vi "initBoardAllInOne.vi"(5 "On Sum\nOff Majority":bool=TRUE, 8 "error in (no error)":errorcluster, 10 "address":string="172.16.7.43", 11 "remote port or service name":u16=9764) -> (0 "error out":errorcluster)   [LabVIEW 2009]
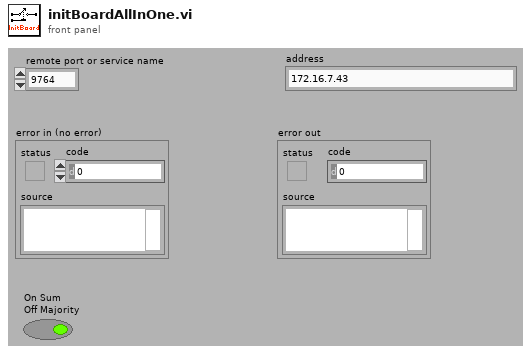
[diagram p1: front panel]
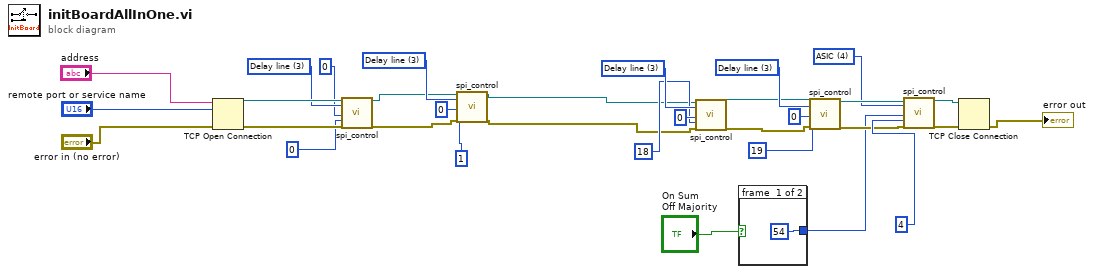
[diagram p0: block diagram]
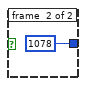
[diagram p2: hidden frame]
diagram:
  w11 = u16 4 items=["Attenuation", "Clipping", "Enable channel", "Delay line", "ASIC"] ("Device")
  w19 = u16 3 items=["Attenuation", "Clipping", "Enable channel", "Delay line", "ASIC"] ("Device")
  w22 = u16 3 items=["Attenuation", "Clipping", "Enable channel", "Delay line", "ASIC"] ("Device")
  w25 = u16 3 items=["Attenuation", "Clipping", "Enable channel", "Delay line", "ASIC"] ("Device")
  w28 = u16 3 items=["Attenuation", "Clipping", "Enable channel", "Delay line", "ASIC"] ("Device")
  n1 = TCP Open Connection(address="address", remote port or service name="remote port or service name", error in (no error)="error in (no error)") -> (connection ID=w29:refnum<k5>, error out=w30:errorcluster)  [unwired: 2 in]
  n2 = call "spi_control.vi"("connection ID"=w29, "Device"=w28, "Data"=0, "Register or channel"=0, "error out 3"=w30) -> ("connection ID out"=w16:refnum<k5>, "error out 2"=w15:errorcluster)  [unwired: 7 in, 6 out]
  n3 = call "spi_control.vi"("connection ID"=w16, "Device"=w25, "Data"=0, "Register or channel"=1, "error out 3"=w15) -> ("connection ID out"=w4:refnum<k5>, "error out 2"=w3:errorcluster)  [unwired: 7 in, 6 out]
  n4 = call "spi_control.vi"("connection ID"=w4, "Device"=w22, "Data"=0, "Register or channel"=18, "error out 3"=w3) -> ("connection ID out"=w14:refnum<k5>, "error out 2"=w13:errorcluster)  [unwired: 7 in, 6 out]
  n5 = case shown="False" "On Sum\nOff Majority" {
    tunnel: [54 ("Data") 1078 ("Data")] -> w2
    frame #0 {
    }
    frame #1 {
    }
  }
  n6 = call "spi_control.vi"("connection ID"=w14, "Device"=w19, "Data"=0, "Register or channel"=19, "error out 3"=w13) -> ("connection ID out"=w12:refnum<k5>, "error out 2"=w9:errorcluster)  [unwired: 7 in, 6 out]
  n7 = call "spi_control.vi"("connection ID"=w12, "Device"=w11, "Data"=w2, "Register or channel"=4, "error out 3"=w9) -> ("connection ID out"=w7:refnum<k5>, "error out 2"=w8:errorcluster)  [unwired: 7 in, 6 out]
  n8 = TCP Close Connection(connection ID=w7, error in (no error)=w8) -> (error out=→"error out":errorcluster)  [unwired: 1 in, 1 out]
